vi "WriteText.vi"(8 "error in (no error)":errorcluster, 9 "Original Input":string, 10 "Picture In":picture, 11 "BarCode in":refnum<class "BarCode.lvclass">) -> (0 "error out":errorcluster, 2 "Picture Out":picture, 3 "BarCode out":refnum<class "BarCode.lvclass">)   [LabVIEW 2013, in "BarCodes.lvlib" / "BarCode.lvclass"]
uses:
  BarCode.lvclass
  BarCode.lvclass/BarCode.ctl
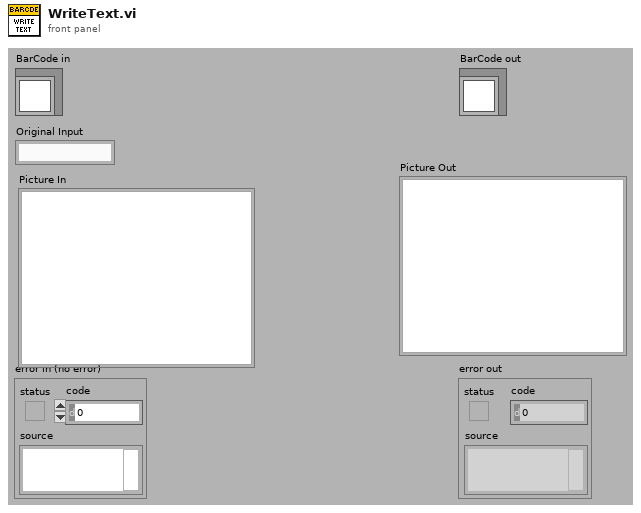
[diagram p1: front panel]
types:
  T1 = enum16{"User-specified Font", "Application Font", "System Font", "Dialog Font"}
  T2 = typedef "BarCodes.lvlib/BarCode.lvclass/TextPosition.ctl" = cluster{"Start Index":u8, "Length":u8, "Text Rectangle":cluster{"left":i16, "top":i16, "right":i16, "bottom":i16}, "Clearing Rect":cluster{"left":i16, "top":i16, "right":i16, "bottom":i16}, "Font":cluster{"Font Name:":string, "Size":i16, "Strikeout?":bool, "Italic?":bool, "Underline?":bool, "Outline?":bool, "Shadow?":bool, "Bold?":bool}}
  T3 = cluster{"left":i16, "top":i16, "right":i16, "bottom":i16}
  T4 = cluster{"Font Name:":string, "Size":i16, "Strikeout?":bool, "Italic?":bool, "Underline?":bool, "Outline?":bool, "Shadow?":bool, "Bold?":bool}
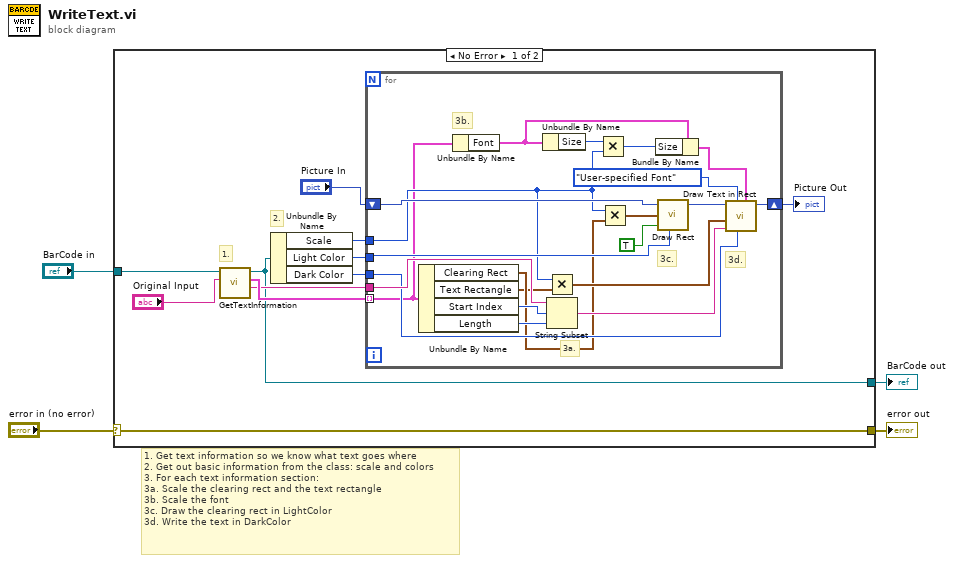
[diagram p0: block diagram]
diagram:
  # "1. Get text information so we know what text goes where\n2. Get out basic information from the class: scale and colors\n3. For each text information section:\n3a. Scale the clearing rect and the text rectangle\n3b. Scale the font\n3c. Draw the clearing rect in LightColor\n3d. Write the text in DarkColor"
  n1 = case shown="No Error" "error in (no error)" {
    selector: "error in (no error)" -> [w15 w38]
    tunnel: [w15 w38] -> w3
    tunnel: [w10 w37] -> w1
    tunnel: "BarCode in" -> [w14 w37]
    frame No Error {
      # "2."
      # "1."
      n2 = call-dynamic "GetTextInformation.vi"("Input"="Original Input", "BarCode in"=w14) -> ("Text"=w11:string, "Text Positions"=w12:T2[], "BarCode out"=w10:refnum<class "BarCode.lvclass">)  [unwired: 6 in, 1 out]
      n3 = Unbundle By Name(w10) -> ("Scale"=w5:u8, "Light Color"=w9:u32, "Dark Color"=w7:u32)
      n4 = for {
        tunnel: w12 -> [w17] mode=indexing
        tunnel: w11 -> [w36]
        tunnel: w9 -> [w35]
        shift-right: [w30] -> w6
        shift-left: "Picture In" -> [w34]
        tunnel: w7 -> [w32]
        tunnel: w5 -> [w24]
        # "3d."
        # "3c."
        # "3b."
        # "3a."
        n5 = Unbundle By Name(w17) -> ("Clearing Rect"=w22:T3, "Text Rectangle"=w21:T3, "Start Index"=w27:u8, "Length"=w26:u8)
        n6 = Unbundle By Name(w17) -> ("Font"=w16:T4)
        n7 = Unbundle By Name(w16) -> ("Size"=w20:i16)
        n8 = Multiply(x=w24, y=w21) -> (x*y=w28:T3)
        n9 = String Subset(string=w36, offset (0)=w27, length (rest)=w26) -> (substring=w31:string)
        n10 = Multiply(x=w20, y=w24) -> (x*y=w19:i16)
        n11 = Multiply(x=w24, y=w22) -> (x*y=w29:T3)
        n12 = Bundle By Name(cluster=w16, "Size"=w19) -> (w23:T4)
        n13 = call <vilib>:"Draw Rect.vi"("picture"=w34, "rect"=w29, "fill?(F)"=TRUE, "color(black)"=w35) -> ("new picture"=w33:picture)  [unwired: 5 in]
        n14 = call <vilib>:"Draw Text in Rect.vi"("[user-specified font]"=w23, "text color(black)"=w32, "desired font(Application)"=T1."User-specified Font", "text"=w31, "rect"=w28, "picture"=w33) -> ("new picture"=w30:picture)  [unwired: 5 in]
      }
      "Picture Out" <- w6
    }
    frame Error {
    }
  }
  "error out" <- w3
  "BarCode out" <- w1
